vi "Initialize.vi"(8 "error in (no error)":errorcluster, 11 "BoardDisplay in":refnum<class "BoardDisplay.lvclass">) -> (0 "error out":errorcluster, 3 "BoardDisplay out":refnum<class "BoardDisplay.lvclass">)   [LabVIEW 2015, in "TronviewPresentation.lvlib" / "BoardDisplay.lvclass"]
uses:
  BoardDisplay.lvclass
  BoardDisplay.lvclass/BoardDisplay.ctl
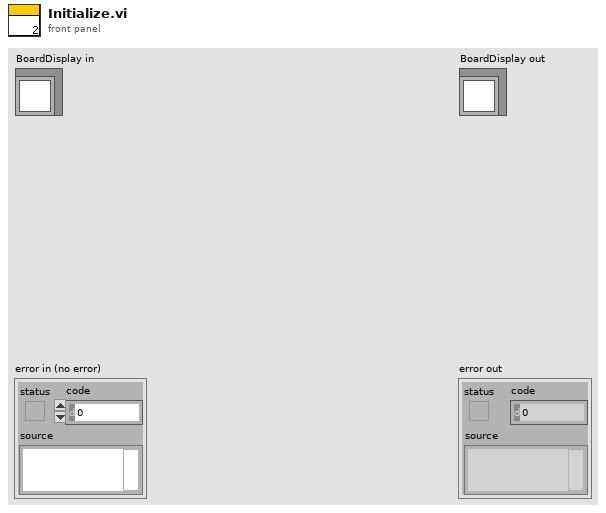
[diagram p1: front panel]
types:
  T1 = typedef "imagedata.ctl" = cluster{"image type":i32, "image depth":i32, "image":u8[], "mask":u8[], "colors":u32[], "Rectangle":cluster{"left":i16, "top":i16, "right":i16, "bottom":i16}}
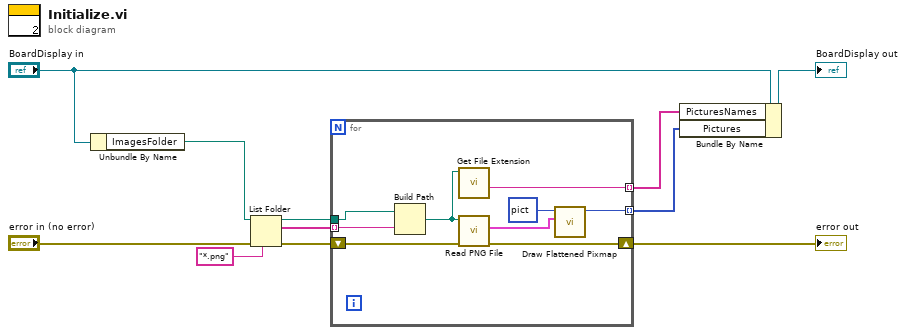
[diagram p0: block diagram]
diagram:
  n1 = Unbundle By Name("BoardDisplay in") -> ("ImagesFolder"=w9:path)
  n2 = List Folder(path=w9, pattern="*.png", error in="error in (no error)") -> (path out=w4:path, filenames=w5:string[], error out=w7:errorcluster)  [unwired: 1 in, 1 out]
  n3 = for {
    shift-right: [w19] -> w6
    shift-left: w7 -> [w20]
    tunnel: w5 -> [w17] mode=indexing
    tunnel: w4 -> [w18]
    tunnel: [w15] -> w2 mode=indexing
    tunnel: [w13] -> w1 mode=indexing
    n4 = Build Path(base path=w18, name or relative path=w17) -> (appended path=w14:path)
    n5 = call <vilib>:"Get File Extension.vi"("file"=w14) -> ("filename without extension"=w13:string)  [unwired: 6 in, 4 out]
    n6 = call <vilib>:"Read PNG File.vi"("error in (no error)"=w20, "path to PNG file"=w14) -> ("error out"=w19:errorcluster, "image data"=w16:T1)  [unwired: 7 in, 1 out]
    n7 = call <vilib>:"Draw Flattened Pixmap.vi"("image data"=w16, "picture"=picture data[5B]) -> ("new picture"=w15:picture)  [unwired: 7 in]
  }
  "error out" <- w6
  n8 = Bundle By Name(cluster="BoardDisplay in", "PicturesNames"=w1, "Pictures"=w2) -> (→"BoardDisplay out":refnum<class "BoardDisplay.lvclass">)
